vi "TTA_MATLAB_Set_Template_Path.vi"(8 "error in":errorcluster, 11 "Template Path":path=path "C:/Users/Alex.Minicozzi.NJ01/Documents/LabVIEW Data/BDS_MATLAB/ViennaGUI") -> (0 "error out":errorcluster)   [LabVIEW 2016]
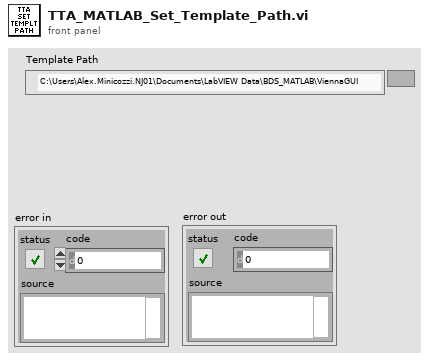
[diagram p1: front panel]
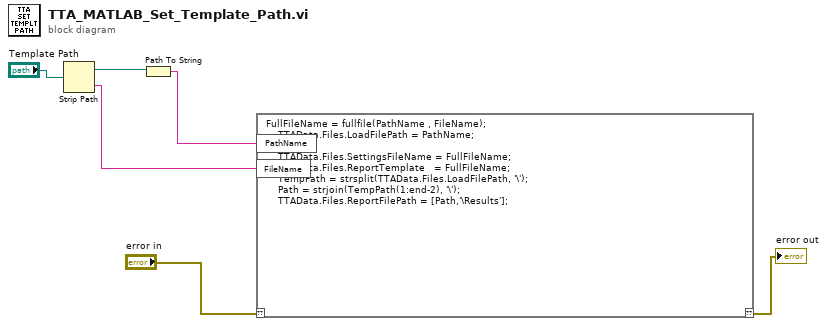
[diagram p0: block diagram]
diagram:
  n1 = Strip Path(path="Template Path") -> (stripped path=w2:path, name=w1:string)
  n2 = Path To String(path=w2) -> (string=w4:string)
  n3 = script code="FullFileName = fullfile(PathName , FileName);\n    TTAData.Files.LoadFilePath = PathName;\n    \n    TTAData.Files.SettingsFileName = FullFileName;\n    TTAData.Files.ReportTemplate   = FullFileName;\n    TempPath = strsplit(TTAData.Files.LoadFilePath, '\\');\n    Path = strjoin(TempPath(1:end-2), '\\');\n    TTAData.Files.ReportFilePath = [Path,'\\Results'];"("??"="error in", "PathName"=w4, "FileName"=w1) -> ("??"=→"error out":errorcluster)
